vi "IsSPCArmed_HH.vi"() -> (0 "Boolean":bool)   [LabVIEW 2009]
uses:
  hhlib.dll
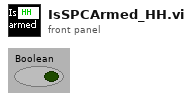
[diagram p1: front panel]
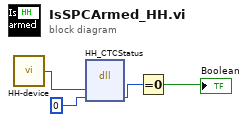
[diagram p0: block diagram]
diagram:
  n1 = call "HH-device.vi"() -> ("Device (output)"=w3:i32)  [unwired: 2 in]
  n2 = dll-call lib="C:/Programme/Anwendungen/DAQLinescan_HH/hhlib.dll" fn="HH_CTCStatus"("devidx"=w3, "ctcstatus"=0) -> ("ctcstatus"=w2:i32)  [unwired: 5 in, 2 out]
  n3 = Equal To 0?(x=w2) -> (x = 0?=→"Boolean":bool)
